vi "Logger-Globals.vi"() -> ()   [LabVIEW 2020]
panel:
  out "Log path":path
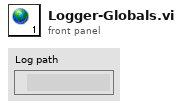
[diagram p1: front panel]
diagram:
